vi "Auto Shift.vi"(9 "Throttle":dbl, 11 "Manual Low Gear":bool) -> (3 "High Gear":bool)   [LabVIEW 2015]
uses:
  Robot Global Data.vi
  Common Code/Auto Shift State.ctl
panel:
  out "Throttle Accel":dbl
  out "Accel":dbl
  out "State":T1=enum."High"
  out "Speed":dbl
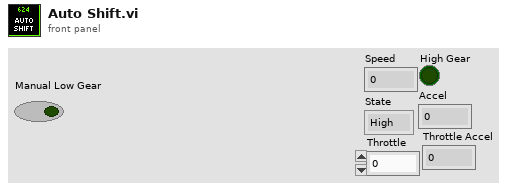
[diagram p1: front panel]
types:
  T1 = typedef "Auto Shift State.ctl" = enum16{"Low", "High"}
  T2 = typedef "Dashboard Control Data.ctl" = cluster{"Encoder Control":T3, "Steer PID output":cluster{"output high":dbl, "output low":dbl}, " Steer PID gains":cluster{"proportional gain (Kc)":dbl, "integral time (Ti, min)":dbl, "derivative time (Td, min)":dbl}, "Drivetrain Settings":T4, "Vision Packet":T5, "Dashboard Drivetrain Command":T6, "Info/Command Cluster":T8, "Ball Vision Packet":T9, "Intake Presets":T11, "Intake Encoder Control":T13, "Climb Presets":T14, "Goal Output Range":cluster{"output high":dbl, "output low":dbl}, "Enabled Systems":T15, "Auton Presets":T16, "Pressure M":dbl, "Pressure B":dbl, "Vision Timeout":dbl, "Auto-Shift":T17, "Catapult Setpoints":T18}
  T3 = typedef "Encoder Control.ctl" = cluster{"Right Tick Constant":dbl, "Left Tick Constant":dbl, "Reset?":bool, "Y Dist":cluster{"PID gains":cluster{"proportional gain (Kc)":dbl, "integral time (Ti, min)":dbl, "derivative time (Td, min)":dbl}}, "Y Stop Thresh":dbl, "Y Stop Speed":dbl}
  T4 = typedef "Drivetrain Settings.ctl" = cluster{"Gyro Tolerance":dbl, "Throttle Ramp (ms)":dbl, "Kv":dbl, "Ka":dbl, "Feed Forward P":dbl, "Feed Forward D":dbl, "Goal Vision PID gains":cluster{"proportional gain (Kc)":dbl, "integral time (Ti, min)":dbl, "derivative time (Td, min)":dbl}, "Goal Detection Window":dbl, "Creep Rate":dbl, "Vision Throttle Threshold":dbl, "Min Turn Output":dbl, "Left Batter Angle":dbl, "Right Batter Angle":dbl}
  T5 = typedef "Goal Vision Packet.ctl" = cluster{"Distance":dbl, "Center X":dbl, "Center Y":dbl, "Found Target?":bool, "Robot Center":dbl, "Angle":dbl}
  T6 = typedef "Dashboard Drivetrain Command.ctl" = cluster{"Drivetrain Vision":T7}
  T7 = typedef "Drivetrain Vision.ctl" = cluster{"Goal Window":dbl, "Ball Window":dbl}
  T8 = typedef "Ball Tracking Command Cluster.ctl" = cluster{"Distance to Ball":dbl, "Desired Angle":dbl, "Command":enum16{"Turn to Ball", "Turn to Angle", "Get Distance"}, "Pixels from Center":dbl}
  T9 = typedef "Ball Vision Packet.ctl" = cluster{"Ball Detected?":bool, "Distance to Ball":dbl, "Desired Angle":dbl, "Pixels from Center":dbl, "Tracking mode":T10}
  T10 = typedef "Tracking Mode.ctl" = enum16{"Turn to Ball", "Turn to Angle"}
  T11 = typedef "Intake Presets.ctl" = cluster{"Intake Speed":dbl, "Outake Speed":dbl, "Angle Speed":dbl, "Angle Tolerance":dbl, "Encoder Scale":dbl, "Load Height":dbl, "Output Range":T12, "MaxCurrent":dbl, "Idle Height":dbl, "Max Height":dbl, "Reset Encoders?":bool, "PID gains":cluster{"proportional gain (Kc)":dbl, "integral time (Ti, min)":dbl, "derivative time (Td, min)":dbl}, "Drop Low Height ":dbl, "Rotation Power Max/Min":dbl}
  T12 = typedef "Drivetrain Output Range.ctl" = cluster{"output high":dbl, "output low":dbl}
  T13 = typedef "IntakeEcoderControl.ctl" = cluster{"Arm Tick Constant":dbl, "Reset?":bool, "Y Dist":cluster{"PID gains":cluster{"proportional gain (Kc)":dbl, "integral time (Ti, min)":dbl, "derivative time (Td, min)":dbl}}, "Y Stop Thresh":dbl, "Y Stop Speed":dbl}
  T14 = typedef "Climb Presets.ctl" = cluster{"Pull Power":dbl, "Extend Power":dbl}
  T15 = typedef "Enabled Systems.ctl" = cluster{"Shoot":bool, "Intake":bool, "DT":bool, "Gyro":bool, "100ms":bool, "US":bool}
  T16 = typedef "Autonomous Presets.ctl" = cluster{"Pitch Limit":dbl, "Roll Limit":dbl, "Start Position":dbl, "Cross Position":dbl}
  T17 = typedef "Auto Shift Cluster.ctl" = cluster{"Delay":dbl, "Speed Thresh":dbl, "Upshift Accel":dbl, "Upshift Throttle":dbl, "Upshift Throttle Accel":dbl, "Downshift Throttle":dbl, "Downshift Throttle Accel":dbl, "Pressure Threshold":dbl}
  T18 = typedef "Catapult Presets.ctl" = cluster{"Intake Danger Height":dbl, "Ball Security Delay ":dbl, "High PSI Minimum":dbl, "Shot Finish Delay":dbl, "Low PSI Minimum":dbl, "Idle Ball Security Wait ":dbl}
  T19 = typedef "Encoder Values Super Cluster.ctl" = cluster{"Left Encoder":T20, "Right Encoder":T20}
  T20 = typedef "Encoder Values.ctl" = cluster{"Distance":dbl, "Speed":dbl, "Ticks":dbl}
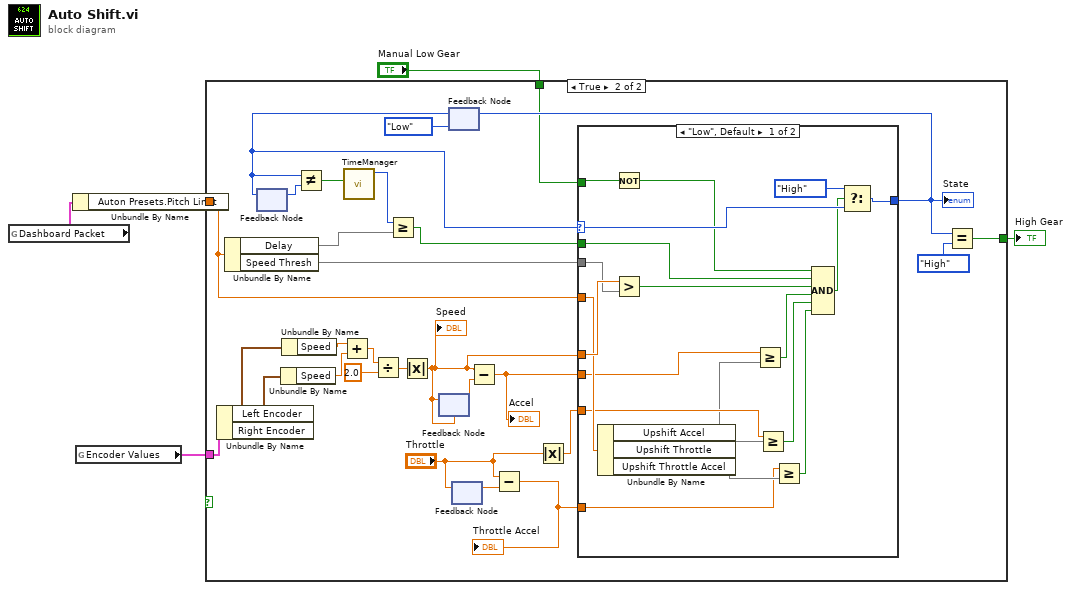
[diagram p0: block diagram]
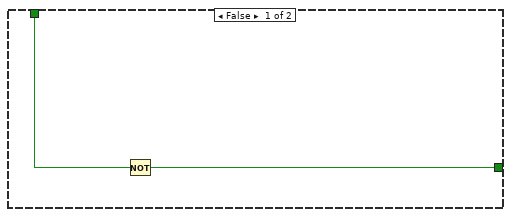
[diagram p2: hidden frame]
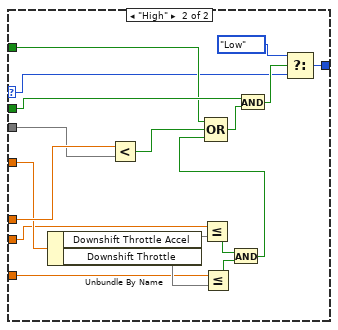
[diagram p3: hidden frame]
diagram:
  n1 = global read "Robot Global Data.vi" "Dashboard Packet"() -> (w6:T2)
  n2 = Unbundle By Name(w6) -> ("Auton Presets.Pitch Limit"=w5:dbl)
  n3 = global read "Robot Global Data.vi" "Encoder Values"() -> (w4:T19)
  n4 = case shown="True" w1 {
    tunnel: w5 -> [_ w13]
    tunnel: w4 -> [_ w36]
    tunnel: [w7 w19] -> w3
    tunnel: "Manual Low Gear" -> [w8 w14]
    frame False {
      n5 = Not(x=w8) -> (.not. x?=w7:bool)
    }
    frame True {
      n6 = Unbundle By Name(w36) -> ("Left Encoder"=w35:T20, "Right Encoder"=w34:T20)
      n7 = Unbundle By Name(w13) -> ("Delay"=w23, "Speed Thresh"=w17)
      n8 = feedback #1() -> (w26:T1)  [unwired: 1 in]
      n9 = Unbundle By Name(w34) -> ("Speed"=w32:dbl)
      n10 = Unbundle By Name(w35) -> ("Speed"=w33:dbl)
      n11 = Add(x=w33, y=w32) -> (x+y=w31:dbl)
      n12 = Divide(x=w31, y=2.0) -> (x/y=w29:dbl)
      n13 = Absolute Value(x=w29) -> (abs(x)=w16:dbl)
      "Speed" <- w16
      n14 = feedback-in #2(w16) -> ()
      n15 = feedback #2(w16) -> (w28:dbl)
      n16 = feedback #3(Auto_Shift_State."Low") -> (w22:T1)
      n17 = feedback-in #1(w22) -> ()
      n18 = Not Equal?(x=w22, y=w26) -> (x != y?=w25:bool)
      n19 = call "TimeManager.vi"("Reset?"=w25) -> ("Time Since Reset"=w24:u32)  [unwired: 9 in, 1 out]
      n20 = Greater Or Equal?(x=w24, y=w23) -> (x >= y?=w21:bool)
      n21 = feedback #4() -> (w12:dbl)  [unwired: 1 in]
      n22 = feedback-in #4("Throttle") -> ()
      n23 = Subtract(x=w16, y=w28) -> (x-y=w15:dbl)
      "Accel" <- w15
      n24 = Subtract(x="Throttle", y=w12) -> (x-y=w9:dbl)
      "Throttle Accel" <- w9
      n25 = Absolute Value(x="Throttle") -> (abs(x)=w10:dbl)
      n26 = case shown="\"Low\", Default" w22 {
        selector: w22 -> [w56 w70]
        tunnel: w21 -> [w51 w72]
        tunnel: [w55 w68] -> w18
        tunnel: w17 -> [w53 w65]
        tunnel: w16 -> [w54 w66]
        tunnel: w15 -> [w40 w60]
        tunnel: w14 -> [w48 w71]
        tunnel: w13 -> [w46 w64]
        tunnel: w10 -> [w42 w62]
        tunnel: w9 -> [w43 _]
        frame "Low", Default {
          n27 = Unbundle By Name(w46) -> ("Upshift Accel"=w41, "Upshift Throttle"=w45, "Upshift Throttle Accel"=w44)
          n28 = Not(x=w48) -> (.not. x?=w47:bool)
          n29 = Greater?(x=w54, y=w53) -> (0:w52:bool)
          n30 = Greater Or Equal?(x=w40, y=w41) -> (x >= y?=w39:bool)
          n31 = Greater Or Equal?(x=w42, y=w45) -> (x >= y?=w38:bool)
          n32 = Greater Or Equal?(x=w43, y=w44) -> (x >= y?=w37:bool)
          n33 = Compound Arithmetic op=AND(w47, w51, w52, w39, w38, w37) -> (w50:bool)
          n34 = Select(t=Auto_Shift_State."High", s=w50, f=w56) -> (s? t:f=w55:T1)
        }
        frame "High" {
          n35 = Unbundle By Name(w64) -> ("Downshift Throttle Accel"=w61, "Downshift Throttle"=w63)
          n36 = Less?(x=w66, y=w65) -> (x < y?=w67:bool)
          n37 = Less Or Equal?(x=w60, y=w61) -> (x <= y?=w59:bool)
          n38 = Less Or Equal?(x=w62, y=w63) -> (x <= y?=w58:bool)
          n39 = And(x=w59, y=w58) -> (x .and. y?=w57:bool)
          n40 = Compound Arithmetic op=OR(w71, w67, w57) -> (w74:bool)
          n41 = And(x=w72, y=w74) -> (x .and. y?=w73:bool)
          n42 = Select(t=Auto_Shift_State."Low", s=w73, f=w70) -> (s? t:f=w68:T1)
        }
      }
      "State" <- w18
      n43 = feedback-in #3(w18) -> ()
      n44 = Equal?(x=w18, y=Auto_Shift_State."High") -> (x = y?=w19:bool)
    }
  }
  "High Gear" <- w3
